vi "Class - ResultCntr.SectionStart.vi"(8 "error in (no error)":errorcluster, 11 "Class - ResultCntr in":refnum<class "Class - ResultCntr.lvclass">) -> (0 "error out":errorcluster, 1 "ID":string, 3 "Class - ResultCntr out":refnum<class "Class - ResultCntr.lvclass">)   [LabVIEW 2017, in "Class - ResultCntr.lvclass"]
uses:
  Class - ResultCntr.lvclass
  Class - ResultCntr.lvclass/Class - ResultCntr.ctl
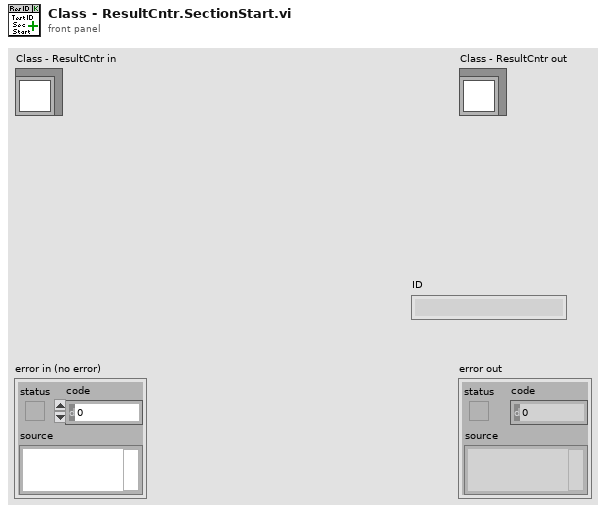
[diagram p1: front panel]
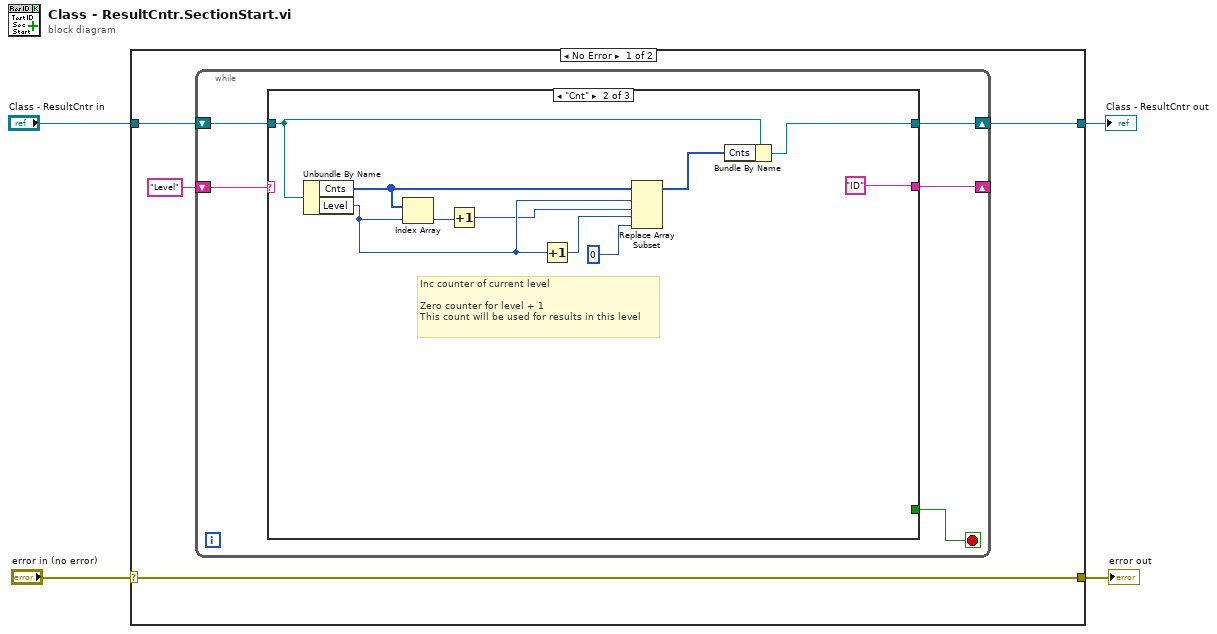
[diagram p0: block diagram]
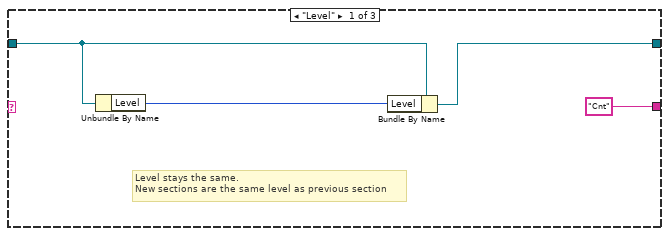
[diagram p2: hidden frame]
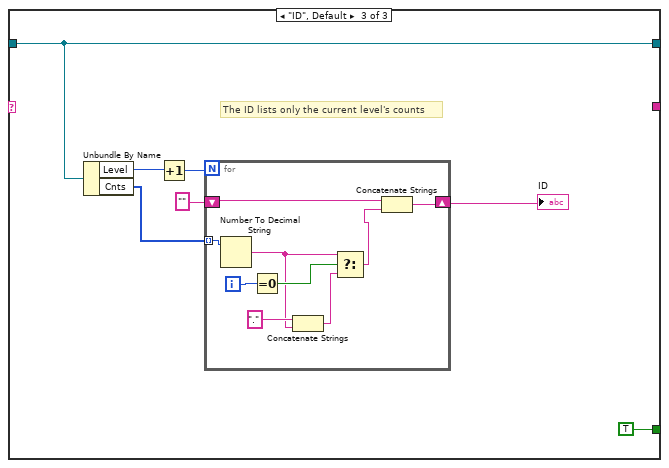
[diagram p3: hidden frame]
diagram:
  n1 = case shown="No Error" "error in (no error)" {
    selector: "error in (no error)" -> [w8 w45]
    tunnel: [w8 w45] -> w3
    tunnel: [w5 w44] -> w1
    tunnel: "Class - ResultCntr in" -> [w7 w44]
    frame No Error {
      n2 = while {
        shift-right: [w11] -> w5
        shift-left: w7 -> [w12]
        shift-right: [w10] -> _
        shift-left: "Level" -> [w13]
        stop <- w9 stop-if-true
        n3 = case shown="\"Cnt\"" w13 {
          tunnel: w12 -> [w15 w25 w31]
          tunnel: [w14 w24 w31] -> w11
          tunnel: ["Cnt" "ID" _] -> w10
          tunnel: [_ _ TRUE] -> w9
          frame "Level" {
            # "Level stays the same.\nNew sections are the same level as previous section"
            n4 = Unbundle By Name(w15) -> ("Level"=w16:i32)
            n5 = Bundle By Name(cluster=w15, "Level"=w16) -> (w14:refnum<class "Class - ResultCntr.lvclass">)
          }
          frame "Cnt" {
            # "Inc counter of current level\n\nZero counter for level + 1\nThis count will be used for results in this level"
            n6 = Unbundle By Name(w25) -> ("Cnts"=w21:i32[], "Level"=w20:i32)
            n7 = Index Array(array=w21, index=w20) -> (element=w19:i32)
            n8 = Increment(x=w19) -> (x+1=w18:i32)
            n9 = Increment(x=w20) -> (x+1=w22:i32)
            n10 = Replace Array Subset(array=w21, new element #1=w18, index #1=w20, new element #2=0 ("new element/subarray"), index #2=w22) -> (w26:i32[])
            n11 = Bundle By Name(cluster=w25, "Cnts"=w26) -> (w24:refnum<class "Class - ResultCntr.lvclass">)
          }
          frame "ID", Default {
            # "The ID lists only the current level's counts"
            n12 = Unbundle By Name(w31) -> ("Level"=w30:i32, "Cnts"=w29:i32[])
            n13 = Increment(x=w30) -> (x+1=w33:i32)
            n14 = for {
              N: w33 -> [_]
              tunnel: w29 -> [w42] mode=indexing
              shift-right: [w37] -> w28
              shift-left: "" -> [w36]
              i -> [w43]
              n15 = Number To Decimal String(number=w42) -> (decimal integer string=w38:string)  [unwired: 1 in]
              n16 = Equal To 0?(x=w43) -> (x = 0?=w39:bool)
              n17 = Concatenate Strings(".", w38) -> (w40:string)
              n18 = Select(t=w38, s=w39, f=w40) -> (s? t:f=w35:string)
              n19 = Concatenate Strings(w36, w35) -> (w37:string)
            }
            "ID" <- w28
          }
        }
      }
    }
    frame Error {
    }
  }
  "error out" <- w3
  "Class - ResultCntr out" <- w1
